vi "Last_modified_date.vi"(0 "Update Now":bool) -> (1 "concatenatedRevisions":string, 2 "localStatus":string)   [LabVIEW 2022 SP3]
uses:
  <vilib>/Utility/error.llb/Trim Whitespace One-Sided.vi
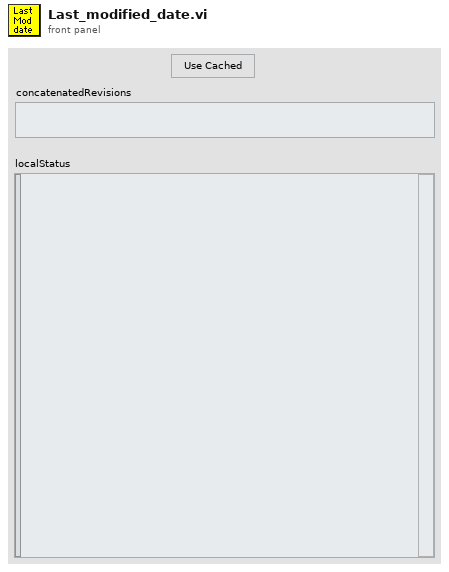
[diagram p1: front panel]
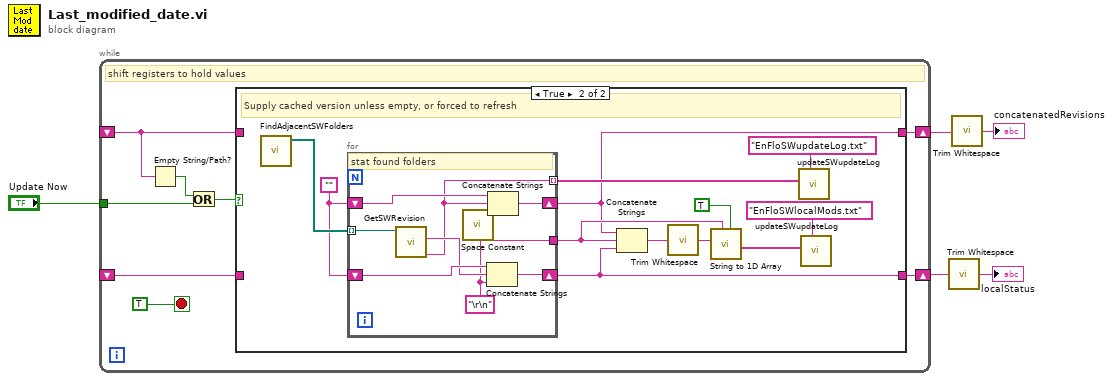
[diagram p0: block diagram]
diagram:
  n1 = while {
    shift-right: [w13] -> w1
    shift-left: _ -> [w9]
    tunnel: "Update Now" -> [w10]
    shift-right: [w7] -> w2
    shift-left: _ -> [w6]
    stop <- TRUE stop-if-true
    # "shift registers to hold values"
    n2 = Empty String/Path?(string/path=w9) -> (empty?=w8:bool)
    n3 = Or(x=w8, y=w10) -> (x .or. y?=w11:bool)
    n4 = case shown="True" w11 {
      tunnel: [w15 w16] -> w13
      tunnel: w9 -> [w15 _]
      tunnel: [w14 w21] -> w7
      tunnel: w6 -> [w14 _]
      frame False {
      }
      frame True {
        w26 = ""
        # "Supply cached version unless empty, or forced to refresh"
        n5 = call "FindAdjacentSWFolders.vi"() -> ("Array"=w27:path[])  [unwired: 10 in, 1 out]
        n6 = for {
          tunnel: w27 -> [w36] mode=indexing
          shift-right: [w29] -> w16
          shift-left: w26 -> [w35]
          shift-right: [w31] -> w21
          shift-left: w26 -> [w33]
          tunnel: [w30] -> w17
          tunnel: [w28] -> w25 mode=indexing
          w30 = "\r\n"
          # "stat found folders"
          n7 = call "GetSWRevision.vi"("File Path Control"=w36) -> ("Brief Output"=w28:string, "localStatus"=w32:string)  [unwired: 8 in, 1 out]
          n8 = call <vilib>:"Space Constant.vi"() -> ("String"=w34:string)
          n9 = Concatenate Strings(w33, w32, w30) -> (w31:string)
          n10 = Concatenate Strings(w35, w28, w34) -> (w29:string)
        }
        n11 = Concatenate Strings(w16, w17, w21) -> (w18:string)
        n12 = call <vilib>:"Trim Whitespace.vi"("string"=w18) -> ("trimmed string"=w19:string)  [unwired: 1 in]
        n13 = call "String to 1D Array.vi"("ignore duplicate delimiters? (F=No)"=TRUE, "delimiter (Tab)"=w17, "String"=w19) -> ("Array of Strings"=w22:string[])  [unwired: 8 in]
        n14 = call "updateSWupdateLog.vi"("name or relative path"="EnFloSWupdateLog.txt", "currentRevisions"=w25) -> ()  [unwired: 10 in]
        n15 = call "updateSWupdateLog.vi"("name or relative path"="EnFloSWlocalMods.txt", "currentRevisions"=w22) -> ()  [unwired: 10 in]
      }
    }
  }
  n16 = call <vilib>:"Trim Whitespace.vi"("string"=w2) -> ("trimmed string"=→"localStatus":string)  [unwired: 1 in]
  n17 = call <vilib>:"Trim Whitespace.vi"("string"=w1) -> ("trimmed string"=→"concatenatedRevisions":string)  [unwired: 1 in]
